vi "CLUSTERSimpleS_A.vi"() -> ()   [LabVIEW 2023]
doc: "This function takes a cluster that contains a DBL, string, and array of I32 (in that order) as input. It squares the value of the DBL, reverses the string, and doubles the value of each element in the array. The result is returned in output.\n\nFor information on the data types used for the DLL function, right-click on the Call Library Function node and choose Configure."
uses:
  CLF_Example.dll
panel:
  out "output":T1
  in  "input":T1={"DBL"=10.0, "String (50 Character Limit)"="abcd", "Array (50 Element Limit)"=[10, 100]}
  # "See the block diagram for more information."
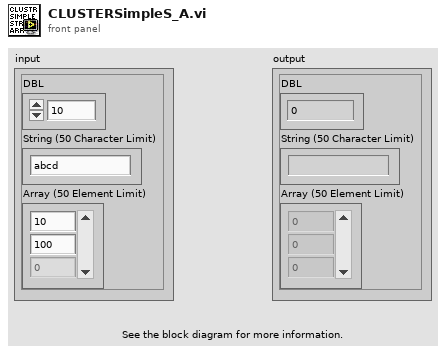
[diagram p1: front panel]
types:
  T1 = cluster{"DBL":dbl, "String (50 Character Limit)":string, "Array (50 Element Limit)":i32[]}
  T2 = cluster{"unsigned byte array[0]":u8, "unsigned byte array[1]":u8, "unsigned byte array[2]":u8, "unsigned byte array[3]":u8, "unsigned byte array[4]":u8, "unsigned byte array[5]":u8, "unsigned byte array[6]":u8, "unsigned byte array[7]":u8, "unsigned byte array[8]":u8, "unsigned byte array[9]":u8, "unsigned byte array[10]":u8, "unsigned byte array[11]":u8, "unsigned byte array[12]":u8, "unsigned byte array[13]":u8, "unsigned byte array[14]":u8, "unsigned byte array[15]":u8, "unsigned byte array[16]":u8, "unsigned byte array[17]":u8, "unsigned byte array[18]":u8, "unsigned byte array[19]":u8, "unsigned byte array[20]":u8, "unsigned byte array[21]":u8, "unsigned byte array[22]":u8, "unsigned byte array[23]":u8, "unsigned byte array[24]":u8, "unsigned byte array[25]":u8, "unsigned byte array[26]":u8, "unsigned byte array[27]":u8, "unsigned byte array[28]":u8, "unsigned byte array[29]":u8, "unsigned byte array[30]":u8, "unsigned byte array[31]":u8, "unsigned byte array[32]":u8, "unsigned byte array[33]":u8, "unsigned byte array[34]":u8, "unsigned byte array[35]":u8, "unsigned byte array[36]":u8, "unsigned byte array[37]":u8, "unsigned byte array[38]":u8, "unsigned byte array[39]":u8, "unsigned byte array[40]":u8, "unsigned byte array[41]":u8, "unsigned byte array[42]":u8, "unsigned byte array[43]":u8, "unsigned byte array[44]":u8, "unsigned byte array[45]":u8, "unsigned byte array[46]":u8, "unsigned byte array[47]":u8, "unsigned byte array[48]":u8, "unsigned byte array[49]":u8, "unsigned byte array[50]":u8}
  T3 = cluster{"Array (50 Element Limit)[0]":i32, "Array (50 Element Limit)[1]":i32, "Array (50 Element Limit)[2]":i32, "Array (50 Element Limit)[3]":i32, "Array (50 Element Limit)[4]":i32, "Array (50 Element Limit)[5]":i32, "Array (50 Element Limit)[6]":i32, "Array (50 Element Limit)[7]":i32, "Array (50 Element Limit)[8]":i32, "Array (50 Element Limit)[9]":i32, "Array (50 Element Limit)[10]":i32, "Array (50 Element Limit)[11]":i32, "Array (50 Element Limit)[12]":i32, "Array (50 Element Limit)[13]":i32, "Array (50 Element Limit)[14]":i32, "Array (50 Element Limit)[15]":i32, "Array (50 Element Limit)[16]":i32, "Array (50 Element Limit)[17]":i32, "Array (50 Element Limit)[18]":i32, "Array (50 Element Limit)[19]":i32, "Array (50 Element Limit)[20]":i32, "Array (50 Element Limit)[21]":i32, "Array (50 Element Limit)[22]":i32, "Array (50 Element Limit)[23]":i32, "Array (50 Element Limit)[24]":i32, "Array (50 Element Limit)[25]":i32, "Array (50 Element Limit)[26]":i32, "Array (50 Element Limit)[27]":i32, "Array (50 Element Limit)[28]":i32, "Array (50 Element Limit)[29]":i32, "Array (50 Element Limit)[30]":i32, "Array (50 Element Limit)[31]":i32, "Array (50 Element Limit)[32]":i32, "Array (50 Element Limit)[33]":i32, "Array (50 Element Limit)[34]":i32, "Array (50 Element Limit)[35]":i32, "Array (50 Element Limit)[36]":i32, "Array (50 Element Limit)[37]":i32, "Array (50 Element Limit)[38]":i32, "Array (50 Element Limit)[39]":i32, "Array (50 Element Limit)[40]":i32, "Array (50 Element Limit)[41]":i32, "Array (50 Element Limit)[42]":i32, "Array (50 Element Limit)[43]":i32, "Array (50 Element Limit)[44]":i32, "Array (50 Element Limit)[45]":i32, "Array (50 Element Limit)[46]":i32, "Array (50 Element Limit)[47]":i32, "Array (50 Element Limit)[48]":i32, "Array (50 Element Limit)[49]":i32}
  T4 = cluster{"DBL":dbl, "unsigned byte array":cluster{"unsigned byte array[0]":u8, "unsigned byte array[1]":u8, "unsigned byte array[2]":u8, "unsigned byte array[3]":u8, "unsigned byte array[4]":u8, "unsigned byte array[5]":u8, "unsigned byte array[6]":u8, "unsigned byte array[7]":u8, "unsigned byte array[8]":u8, "unsigned byte array[9]":u8, "unsigned byte array[10]":u8, "unsigned byte array[11]":u8, "unsigned byte array[12]":u8, "unsigned byte array[13]":u8, "unsigned byte array[14]":u8, "unsigned byte array[15]":u8, "unsigned byte array[16]":u8, "unsigned byte array[17]":u8, "unsigned byte array[18]":u8, "unsigned byte array[19]":u8, "unsigned byte array[20]":u8, "unsigned byte array[21]":u8, "unsigned byte array[22]":u8, "unsigned byte array[23]":u8, "unsigned byte array[24]":u8, "unsigned byte array[25]":u8, "unsigned byte array[26]":u8, "unsigned byte array[27]":u8, "unsigned byte array[28]":u8, "unsigned byte array[29]":u8, "unsigned byte array[30]":u8, "unsigned byte array[31]":u8, "unsigned byte array[32]":u8, "unsigned byte array[33]":u8, "unsigned byte array[34]":u8, "unsigned byte array[35]":u8, "unsigned byte array[36]":u8, "unsigned byte array[37]":u8, "unsigned byte array[38]":u8, "unsigned byte array[39]":u8, "unsigned byte array[40]":u8, "unsigned byte array[41]":u8, "unsigned byte array[42]":u8, "unsigned byte array[43]":u8, "unsigned byte array[44]":u8, "unsigned byte array[45]":u8, "unsigned byte array[46]":u8, "unsigned byte array[47]":u8, "unsigned byte array[48]":u8, "unsigned byte array[49]":u8, "unsigned byte array[50]":u8}, "Array (50 Element Limit)":cluster{"Array (50 Element Limit)[0]":i32, "Array (50 Element Limit)[1]":i32, "Array (50 Element Limit)[2]":i32, "Array (50 Element Limit)[3]":i32, "Array (50 Element Limit)[4]":i32, "Array (50 Element Limit)[5]":i32, "Array (50 Element Limit)[6]":i32, "Array (50 Element Limit)[7]":i32, "Array (50 Element Limit)[8]":i32, "Array (50 Element Limit)[9]":i32, "Array (50 Element Limit)[10]":i32, "Array (50 Element Limit)[11]":i32, "Array (50 Element Limit)[12]":i32, "Array (50 Element Limit)[13]":i32, "Array (50 Element Limit)[14]":i32, "Array (50 Element Limit)[15]":i32, "Array (50 Element Limit)[16]":i32, "Array (50 Element Limit)[17]":i32, "Array (50 Element Limit)[18]":i32, "Array (50 Element Limit)[19]":i32, "Array (50 Element Limit)[20]":i32, "Array (50 Element Limit)[21]":i32, "Array (50 Element Limit)[22]":i32, "Array (50 Element Limit)[23]":i32, "Array (50 Element Limit)[24]":i32, "Array (50 Element Limit)[25]":i32, "Array (50 Element Limit)[26]":i32, "Array (50 Element Limit)[27]":i32, "Array (50 Element Limit)[28]":i32, "Array (50 Element Limit)[29]":i32, "Array (50 Element Limit)[30]":i32, "Array (50 Element Limit)[31]":i32, "Array (50 Element Limit)[32]":i32, "Array (50 Element Limit)[33]":i32, "Array (50 Element Limit)[34]":i32, "Array (50 Element Limit)[35]":i32, "Array (50 Element Limit)[36]":i32, "Array (50 Element Limit)[37]":i32, "Array (50 Element Limit)[38]":i32, "Array (50 Element Limit)[39]":i32, "Array (50 Element Limit)[40]":i32, "Array (50 Element Limit)[41]":i32, "Array (50 Element Limit)[42]":i32, "Array (50 Element Limit)[43]":i32, "Array (50 Element Limit)[44]":i32, "Array (50 Element Limit)[45]":i32, "Array (50 Element Limit)[46]":i32, "Array (50 Element Limit)[47]":i32, "Array (50 Element Limit)[48]":i32, "Array (50 Element Limit)[49]":i32}}
  T5 = cluster{"DBL":dbl, "string":string, "Array (50 Element Limit)":i32[]}
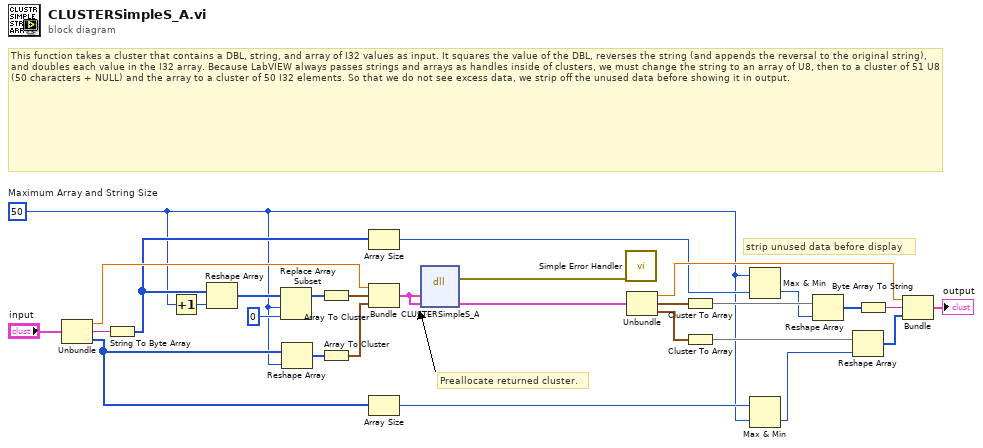
[diagram p0: block diagram]
diagram:
  w1 = 50  # Maximum Array and String Size
  # "strip unused data before display"
  # "Preallocate returned cluster."
  # "This function takes a cluster that contains a DBL, string, and array of I32 values as input. It squares the value of the DBL, reverses the string (and appends the reversal to the original string), and doubles each value in the I32 array. Because LabVIEW always passes strings and arrays as handles inside of clusters, we must change the string to an array of U8, then to a cluster of 51 U8 (50 characters + NULL) and the array to a cluster of 50 I32 elements. So that we do not see excess data, we strip off the unused data before showing it in output."
  n1 = Unbundle("input") -> ("DBL"=w13:dbl, "String (50 Character Limit)"=w18:string, "Array (50 Element Limit)"=w29:i32[])
  n2 = String To Byte Array(string=w18) -> (unsigned byte array=w9:u8[])
  n3 = Increment(x=w1) -> (x+1=w2:i32)
  n4 = Reshape Array(w9, w2) -> (w17:u8[])
  n5 = Replace Array Subset(array=w17, new element=u8 0 ("new element/subarray"), index=w1) -> (w15:u8[])
  n6 = Reshape Array(w29, w1) -> (w16:i32[])
  n7 = Array To Cluster(array=w15) -> (cluster=w14:T2)
  n8 = Array To Cluster(array=w16) -> (cluster=w12:T3)
  n9 = Array Size(array=w9) -> (size(s)=w4:i32)
  n10 = Bundle("DBL"=w13, "unsigned byte array"=w14, "Array (50 Element Limit)"=w12) -> (w11:T4)  [unwired: 1 out]
  n11 = Array Size(array=w29) -> (size(s)=w6:i32)
  n12 = dll-call lib="c:/dev/_r/4/eng/lv-core/lvpostprocessingd/lv_mc_x86_64/dist_i386/examples/Connectivity/Libraries and Executables/DLL Calling VIs/CLF_Example**.*" fn="CLUSTERSimpleS_A"("input"=w11, "output"=w11) -> (error out=w3:errorcluster, "output"=w28:T4)  [unwired: 3 in, 3 out]
  n13 = call <vilib>:"Simple Error Handler.vi"("error in (no error)"=w3) -> ()  [unwired: 4 in, 5 out]
  n14 = Unbundle(w28) -> ("DBL"=w25:dbl, "unsigned byte array"=w22:T2, "Array (50 Element Limit)"=w23:T3)
  n15 = Cluster To Array(cluster=w22) -> (array=w10:u8[])
  n16 = Cluster To Array(cluster=w23) -> (array=w27:i32[])
  n17 = Max & Min(x=w1, y=w4) -> (min(x,y)=w5:i32)  [unwired: 1 out]
  n18 = Max & Min(x=w6, y=w1) -> (min(x,y)=w7:i32)  [unwired: 1 out]
  n19 = Reshape Array(w10, w5) -> (w8:u8[])
  n20 = Reshape Array(w27, w7) -> (w24:i32[])
  n21 = Byte Array To String(unsigned byte array=w8) -> (string=w21:string)
  n22 = Bundle("DBL"=w25, "string"=w21, "Array (50 Element Limit)"=w24) -> (→"output":T5)  [unwired: 1 out]
